vi "Read variant from file.vi"(8 "error in (no error)":errorcluster, 10 "group name in":string, 11 "tdms file":refnum<k34>) -> (0 "error out":errorcluster, 1 "variant out":variant, 3 "tdms file out":refnum<k34>)   [LabVIEW 2015]
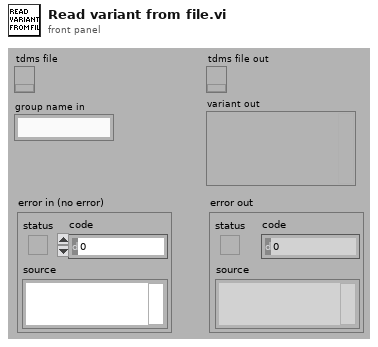
[diagram p1: front panel]
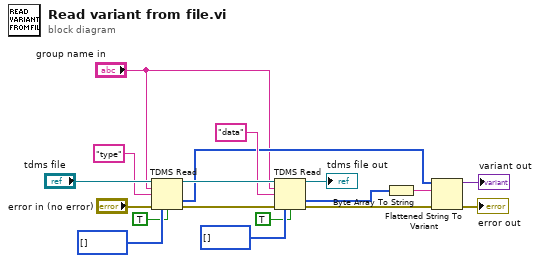
[diagram p0: block diagram]
diagram:
  n1 = TDMS Read(0:"tdms file", 5:"group name in", 7:"type", 11:"error in (no error)", 12:i16[] [] ("type string"), 13:TRUE ("return channels in file order? (F)")) -> (4:w16:refnum<k34>, 10:w12:i16[], 15:w4:errorcluster)  [unwired: 2 in, 3 out]
  n2 = TDMS Read(0:w16, 5:"group name in", 7:"data", 11:w4, 12:u8[] [], 13:TRUE ("return channels in file order? (F)")) -> (4:→"tdms file out":refnum<k34>, 10:w9:u8[], 15:w3:errorcluster)  [unwired: 2 in, 3 out]
  n3 = Byte Array To String(unsigned byte array=w9) -> (string=w10:string)
  n4 = Flattened String To Variant(4:w3, 6:w10, 7:w12) -> (0:→"error out":errorcluster, 3:→"variant out":variant)
